vi "Tool.Dots.vi"(10 "Dot Settings":refnum<class "Dot Settings.lvclass">[](array[class]), 11 "Dots":refnum<class "Dot.lvclass">[](array[class])) -> (3 "Commands":T2(array[cluster]))   [LabVIEW 2019]
uses:
  Classes/Parse/Dot/Dot.lvclass
  <userlib>/LevyLab/Relay Box/Typedefs/Resistor--enum.ctl
  Classes/Settings/Dot Settings/Dot Settings.lvclass
  C:/Users/Albro/Documents/GitHub/AFM-Lithography/lvsrc/Classes/Settings/ObjectSettings/ObjectSettings.lvclass
  Classes/Parse/Dot/Dot.lvclass/Dot.ctl
  Classes/Settings/Dot Settings/Dot Settings.lvclass/Dot Settings.ctl
  Classes/Settings/ObjectSettings/ObjectSettings.lvclass/ObjectSettings.ctl
  Classes/Settings/ObjectSettings/Accessors/Read Enabled.vi
  Classes/Parse/Dot/Read cx.vi
  Classes/Parse/Dot/Read cy.vi
  Global Variables.vi
  <userlib>/LevyLab/Relay Box/Relay-Box.lvclass
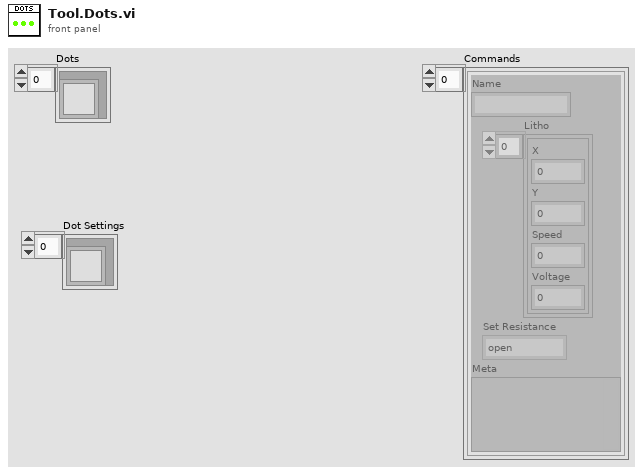
[diagram p1: front panel]
types:
  T1 = typedef "Relay-Box.lvclass/Resistor--enum.ctl" = enum16{"open", "discharge tip", "0 ohms", "100k ohm", "10M ohm", "1G ohm"}
  T2 = cluster{"Name":string, "Litho":cluster{"X":dbl, "Y":dbl, "Speed":dbl, "Voltage":dbl}[], "Set Resistance":T1, "Meta":variant}[]
  T3 = cluster{"X":dbl, "Y":dbl, "Speed":dbl, "Voltage":dbl}[]
  T4 = cluster{"Name":string, "Litho":cluster{"X":dbl, "Y":dbl, "Speed":dbl, "Voltage":dbl}[], "Set Resistance":T1, "Meta":variant}
  T5 = cluster{"X":dbl, "Y":dbl, "Speed":dbl, "Voltage":dbl}
  T6 = typedef "Dot Settings.lvclass/Action.ctl" = enum16{"IV", "QD"}
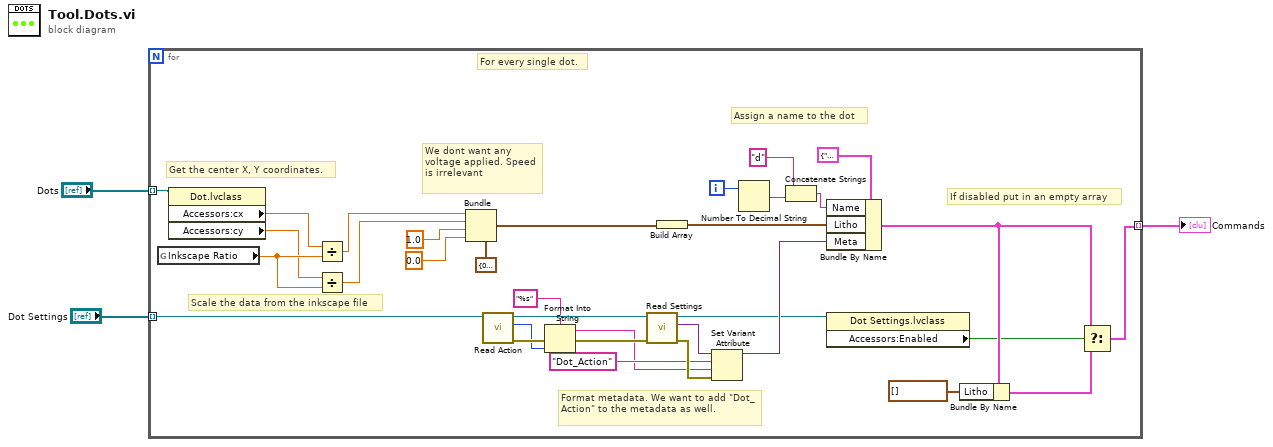
[diagram p0: block diagram]
diagram:
  n1 = for {
    tunnel: "Dots" -> [w36] mode=indexing
    tunnel: [w11] -> w2 mode=indexing
    tunnel: "Dot Settings" -> [w15] mode=indexing
    i -> [w35]
    # "If disabled put in an empty array"
    # "For every single dot."
    # "Get the center X, Y coordinates."
    # "Assign a name to the dot"
    # "Format metadata. We want to add \"Dot_Action\" to the metadata as well."
    # "We dont want any voltage applied. Speed is irrelevant"
    # "Scale the data from the inkscape file"
    n2 = global read "Global Variables.vi" "Inkscape Ratio"() -> (w18:dbl)
    n3 = property class="Dot.lvclass"(reference=w36) -> ("Accessors:cx"=w20:dbl, "Accessors:cy"=w17:dbl)  [unwired: 1 in, 2 out]
    n4 = Divide(x=w20, y=w18) -> (x/y=w19:dbl)
    n5 = Divide(x=w17, y=w18) -> (x/y=w16:dbl)
    n6 = Bundle(cluster=T5 {"X"=0.0, "Y"=0.0, "Speed"=0.0, "Voltage"=0.0} ("Litho Point"), "X"=w19, "Y"=w16, "Speed"=1.0, "Voltage"=0.0) -> (w21:T5)
    n7 = call "Read Action.vi"("Dot Settings in"=w15) -> ("error out"=w8:errorcluster, "Action"=w5:T6, "Dot Settings out"=w25:refnum<class "Dot Settings.lvclass">)  [unwired: 8 in]
    n8 = Format Into String(format string="%s", error in=w8, w5) -> (resulting string=w4:string, error out=w7:errorcluster)  [unwired: 1 in]
    n9 = call "Read Settings.vi"("error in (no error)"=w7, "Dot Settings in"=w25) -> ("error out"=w24:errorcluster, "Settings"=w22:variant, "Dot Settings out"=w9:refnum<class "Dot Settings.lvclass">)  [unwired: 7 in]
    n10 = Build Array(w21) -> (w27:T3)
    n11 = Set Variant Attribute(Variant=w22, name="Dot_Action", value=w4, error in=w24) -> (Variant out=w26:variant)  [unwired: 2 out]
    n12 = Number To Decimal String(number=w35) -> (decimal integer string=w34:string)  [unwired: 1 in]
    n13 = Concatenate Strings("d" ("Name"), w34) -> (w29:string)
    n14 = Bundle By Name(cluster=T4 {"Name"="", "Litho"=[], "Set Resistance"=enum."open", "Meta"=variant} ("Pattern Data"), "Name"=w29, "Litho"=w27, "Meta"=w26) -> (w12:T4)
    n15 = property class="Dot Settings.lvclass"(reference=w9) -> ("Accessors:Enabled"=w10:bool)  [unwired: 1 in, 2 out]
    n16 = Bundle By Name(cluster=w12, "Litho"=T3 []) -> (w13:T4)
    n17 = Select(t=w12, s=w10, f=w13) -> (s? t:f=w11:T4)
  }
  "Commands" <- w2
